vi "nivsfpga_UniqueModName.vi"(1 "String In":string, 2 "Strings":string[](array[string])) -> (0 "Unique String Out":string)   [LabVIEW 2010]
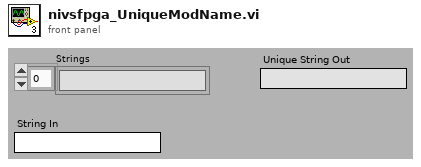
[diagram p1: front panel]
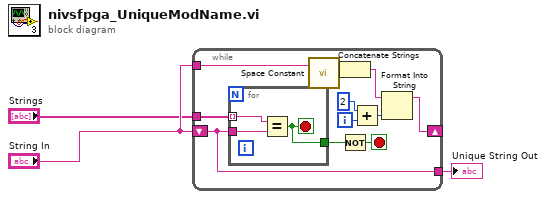
[diagram p0: block diagram]
diagram:
  n1 = while {
    tunnel: "Strings" -> [w14]
    shift-right: [w8] -> _
    shift-left: "String In" -> [w5]
    tunnel: [w5] -> w3
    tunnel: "String In" -> [w6]
    i -> [w12]
    stop <- w13 stop-if-true
    n2 = for {
      tunnel: w14 -> [w17] mode=indexing
      tunnel: w5 -> [w16]
      tunnel: [w15] -> w10
      stop <- w15 stop-if-true
      n3 = Equal?(x=w17, y=w16) -> (x = y?=w15:bool)
    }
    n4 = call <vilib>:"Space Constant.vi"() -> ("String"=w4:string)
    n5 = Concatenate Strings(w6, w4) -> (w7:string)
    n6 = Not(x=w10) -> (.not. x?=w13:bool)
    n7 = Add(x=2, y=w12) -> (x+y=w9:i32)
    n8 = Format Into String(initial string=w7, w9) -> (resulting string=w8:string)  [unwired: 2 in, 1 out]
  }
  "Unique String Out" <- w3
